vi "scratch.vi"() -> ()   [LabVIEW 2017, in "LVJSON.lvlib"]
uses:
  LVJSON.lvlib
  JSON Parsing/Token Types.ctl
  JSON Data Classes/JSON String/JSON String.lvclass
  C:/Users/tblair/Documents/Git Projects/LVJSON/JSON Data Classes/JSON Datatype/JSON Datatype.lvclass
  JSON Data Classes/JSON Numeric/JSON Numeric.lvclass
  JSON Data Classes/JSON Boolean/JSON Boolean.lvclass
  JSON Data Classes/JSON Null/JSON Null.lvclass
  JSON Data Classes/JSON Array/JSON Array.lvclass
  JSON Data Classes/JSON Object/JSON Object.lvclass
  JSON Data Classes/JSON Boolean/New JSON Boolean.vi
  JSON Data Classes/JSON String/New JSON String.vi
  JSON Data Classes/JSON Array/New JSON Array (Numeric).vi
  JSON Data Classes/JSON Object/New JSON Object.vi
  JSON Data Classes/JSON Null/New JSON Null.vi
  JSON Data Classes/JSON Object/Insert Key Value Pair (Single).vi
  JSON Data Classes/JSON Object/Insert Key Value Pair (Multi).vi
  JSON Data Classes/JSON Array/New JSON Array (JSON Data).vi
  JSON Data Classes/JSON Datatype/JSON Datatype.lvclass
  C:/Users/tblair/Documents/Git Projects/LVJSON/JSON Data Classes/JSON Basic Type/JSON Basic Type.lvclass
panel:
  out "Tokens":cluster{"Token Type":T1, "Token Value":string}[](array[cluster])
  out "error out":errorcluster
  out "Object string":string
  out "Object string out":string
  out "Array string out":string
  out "array w/ subset deleted":cluster{"Token Type":T1, "Token Value":string}[](array[cluster])
  out "Array string":string
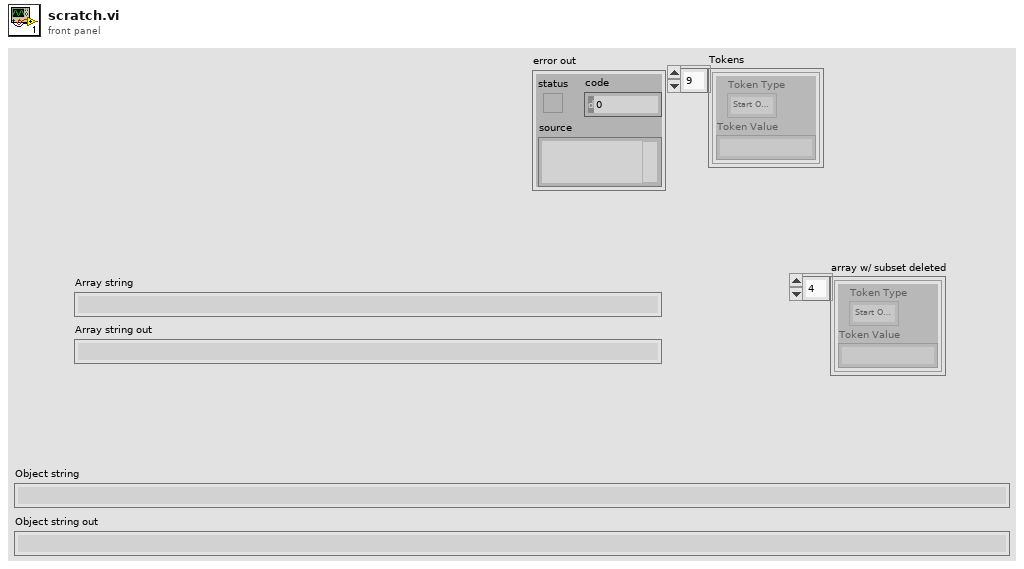
[diagram p1: front panel]
types:
  T1 = typedef "Token Types.ctl" = enum32{"Start Object", "End Object", "Start Array", "End Array", "Colon", "Comma", "Numeric", "true", "false", "null", "String"}
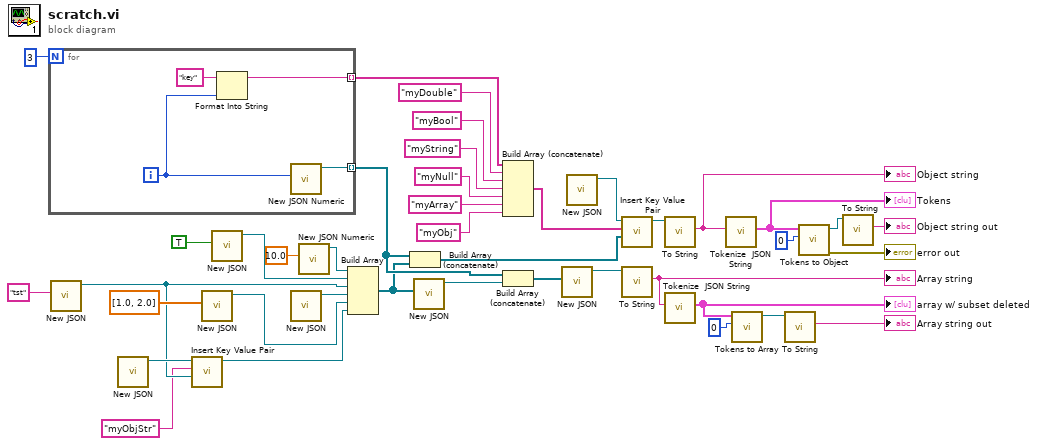
[diagram p0: block diagram]
diagram:
  n1 = for {
    N: 3 -> [_]
    tunnel: [w44] -> w16 mode=indexing
    tunnel: [w41] -> w24 mode=indexing
    i -> [w43]
    n2 = Format Into String(initial string="key", w43) -> (resulting string=w41:string)  [unwired: 2 in, 1 out]
    n3 = call "New JSON Numeric.vi"("value"=w43) -> ("JSON String out"=w44:refnum<class "JSON Numeric.lvclass">)  [unwired: 9 in, 1 out]
  }
  n4 = call-poly "New JSON.vi"("value"="tst") -> ("JSON String out"=w4:refnum<class "JSON String.lvclass">)  [unwired: 9 in, 1 out]
  n5 = call-poly "New JSON.vi"() -> ("JSON Object out"=w5:refnum<class "JSON Object.lvclass">)  [unwired: 10 in, 1 out]
  n6 = call-poly "Insert Key Value Pair.vi"("value"=w4, "key"="myObjStr", "JSON Object in"=w5) -> ("JSON Object out"=w2:refnum<class "JSON Object.lvclass">)  [unwired: 7 in, 1 out]
  n7 = call-poly "New JSON.vi"("Numeric Array"=dbl[] [1.0, 2.0]) -> ("JSON Array out"=w6:refnum<class "JSON Array.lvclass">)  [unwired: 9 in, 1 out]
  n8 = call-poly "New JSON.vi"("value"=TRUE) -> ("JSON String out"=w36:refnum<class "JSON Boolean.lvclass">)  [unwired: 9 in, 1 out]
  n9 = call-poly "New JSON.vi"() -> ("JSON String out"=w17:refnum<class "JSON Null.lvclass">)  [unwired: 10 in, 1 out]
  n10 = call "New JSON Numeric.vi"("value"=10.0) -> ("JSON String out"=w37:refnum<class "JSON Numeric.lvclass">)  [unwired: 9 in, 1 out]
  n11 = Build Array(w37, w36, w4, w17, w6, w2) -> (w15:refnum<class "JSON Datatype.lvclass">[])
  n12 = Build Array (concatenate)(w16, w15) -> (w14:refnum<class "JSON Datatype.lvclass">[])
  n13 = call-poly "New JSON.vi"("Boolean Array"=w15) -> ("JSON Array out"=w34:refnum<class "JSON Array.lvclass">)  [unwired: 9 in, 1 out]
  n14 = Build Array (concatenate)(w24, "myDouble", "myBool", "myString", "myNull", "myArray" ("element"), "myObj" ("element")) -> (w19:string[])
  n15 = Build Array (concatenate)(w16, w34) -> (w33:refnum<class "JSON Datatype.lvclass">[])
  n16 = call-poly "New JSON.vi"("Boolean Array"=w33) -> ("JSON Array out"=w8:refnum<class "JSON Array.lvclass">)  [unwired: 9 in, 1 out]
  n17 = call-poly "New JSON.vi"() -> ("JSON Object out"=w31:refnum<class "JSON Object.lvclass">)  [unwired: 10 in, 1 out]
  n18 = call-poly "Insert Key Value Pair.vi"("values"=w14, "keys"=w19, "JSON Object in"=w31) -> ("JSON Object out"=w30:refnum<class "JSON Object.lvclass">)  [unwired: 7 in, 1 out]
  n19 = call-dynamic "To String.vi"("JSON Array in"=w8) -> ("String"=w35:string)  [unwired: 10 in]
  "Array string" <- w35
  n20 = call-dynamic "To String.vi"("JSON Object in"=w30) -> ("String"=w25:string)  [unwired: 10 in]
  "Object string" <- w25
  n21 = call "Tokenize  JSON String.vi"("JSON String"=w35) -> ("Value Tokens"=w10:cluster{"Token Type":T1, "Token Value":string}[])  [unwired: 10 in]
  "array w/ subset deleted" <- w10
  n22 = call "Tokenize  JSON String.vi"("JSON String"=w25) -> ("Value Tokens"=w29:cluster{"Token Type":T1, "Token Value":string}[])  [unwired: 10 in]
  "Tokens" <- w29
  n23 = call "Tokens to Array.vi"("starting index"=0, "array w/ subset deleted"=w10) -> ("JSON Array out"=w13:refnum<class "JSON Array.lvclass">)  [unwired: 7 in, 2 out]
  n24 = call-dynamic "To String.vi"("JSON Array in"=w13) -> ("String"=→"Array string out":string)  [unwired: 10 in]
  n25 = call "Tokens to Object.vi"("starting index"=0, "array w/ subset deleted"=w29) -> ("error out"=→"error out":errorcluster, "JSON Object out"=w27:refnum<class "JSON Object.lvclass">)  [unwired: 7 in, 1 out]
  n26 = call-dynamic "To String.vi"("JSON Object in"=w27) -> ("String"=→"Object string out":string)  [unwired: 10 in]
